vi "Set Name.vi"(8 "error in (no error)":errorcluster, 10 "Name('')":string, 11 "Admin_Actor in":refnum<class "Admin_Actor.lvclass">) -> (0 "error out":errorcluster, 3 "Admin_Actor out":refnum<class "Admin_Actor.lvclass">)   [LabVIEW 2015]
uses:
  Admin_Actor.lvclass
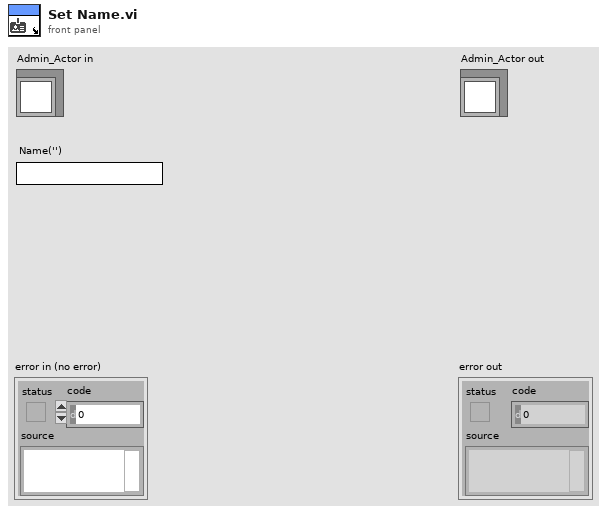
[diagram p1: front panel]
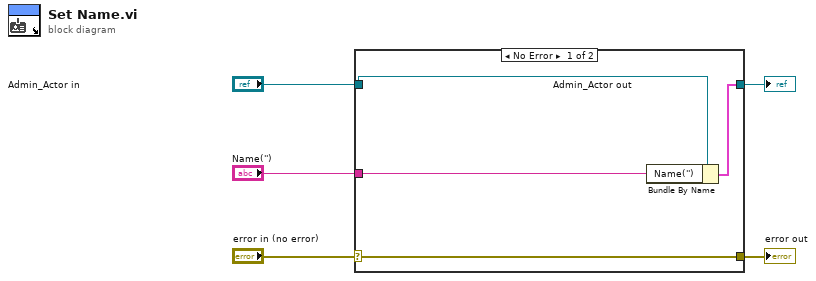
[diagram p0: block diagram]
diagram:
  n1 = case shown="No Error" "error in (no error)" {
    selector: "error in (no error)" -> [w9 w10]
    tunnel: [w9 w10] -> w4
    tunnel: [w7 w11] -> w2
    tunnel: "Admin_Actor in" -> [w8 w11]
    tunnel: "Name('')" -> [w6 _]
    frame No Error {
      n2 = Bundle By Name(cluster=w8, "Name('')"=w6) -> (w7:cluster{})
    }
    frame Error {
    }
  }
  "error out" <- w4
  "Admin_Actor out" <- w2
